vi "01到0-1.vi"(1 "1,0码元":i8[](array[numeric])) -> (0 "1，-1码元":i8[](array[numeric]))   [LabVIEW 2013]
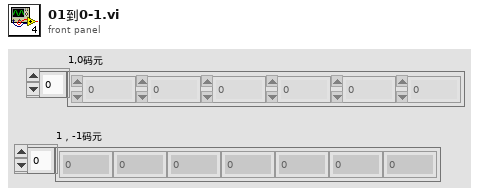
[diagram p1: front panel]
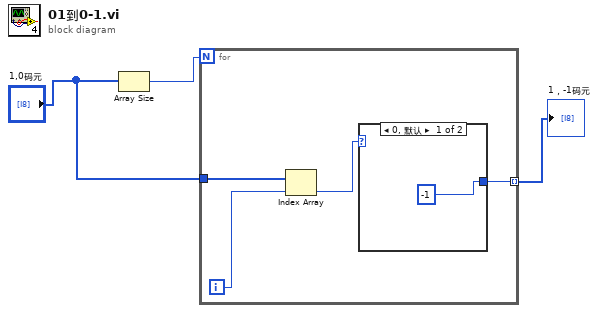
[diagram p0: block diagram]
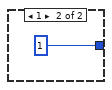
[diagram p2: hidden frame]
diagram:
  n1 = Array Size(array="1,0码元") -> (size(s)=w2:i32)
  n2 = for {
    N: w2 -> [_]
    tunnel: [w7] -> w3 mode=indexing
    tunnel: "1,0码元" -> [w6]
    i -> [w5]
    n3 = Index Array(array=w6, index=w5) -> (element=w4:i8)
    n4 = case shown="0, 默认" w4 {
      tunnel: [-1 1] -> w7
      frame 0, Default {
      }
      frame 1 {
      }
    }
  }
  "1，-1码元" <- w3
